vi "Ctrlr 2 Flag.vi"(8 "AutoArmIn":u8, 10 "Controller in":string, 11 "Enabled?":enum16{"Disabled", "Enabled"}(ring)) -> (0 "AutoArm Out":u8)   [LabVIEW 2012, in "BlockParty4150.lvrbt"]
uses:
  BlockParty4150.lvrbt
  <vilib>/NXT/Hardware/Plugins/Tetrix DC Motor/TetrixDCMotorAddress.ctl
  <vilib>/NXT/Hardware/Plugins/Tetrix 180 deg Servo/Tetrix180ServoAddress.ctl
  <vilib>/FTC/FTC Calculate Drive Power - Tank.vi
  <vilib>/NXT/NXTIO Xnodes/NXTIONodeSubVIs/TETRIX IO Move DC Motors.vi
  <vilib>/NXT/NXTIO Xnodes/NXTIONodeSubVIs/TETRIX IO Move Servos.vi
  <vilib>/NXT/NXTIO Xnodes/AddressXNode/NXTIOAddress.xnode
  <vilib>/NXT/Subs/LVHSConnector.ctl
  <vilib>/NXT/NXTIO Xnodes/NXTIOXNode/NXTIO.xnode
  <vilib>/NXT/LegoClasses/BrickReference/BrickReference.lvclass
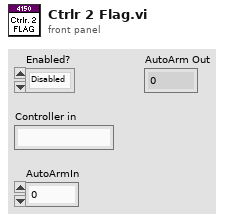
[diagram p1: front panel]
types:
  T1 = typedef "FTC ControllerState.ctl" = cluster{"Left X":i8, "Left Y":i8, "Right X":i8, "Right Y":i8, "Button Encoding 9-12":u8, "Button Encoding 1-8":u8, "POV":T2}
  T2 = typedef "FTC POVState.ctl" = i8
  T3 = typedef "FTC ButtonState.ctl" = cluster{"Button 1":bool, "Button 2":bool, "Button 3":bool, "Button 4":bool, "Button 5":bool, "Button 6":bool, "Button 7":bool, "Button 8":bool, "Button 9":bool, "Button 10":bool, "Button 11":bool, "Button 12":bool, "POV":T2}
  T4 = typedef "TetrixDCMotorAddress.ctl" = i32
  T5 = typedef "Tetrix180ServoAddress.ctl" = i32
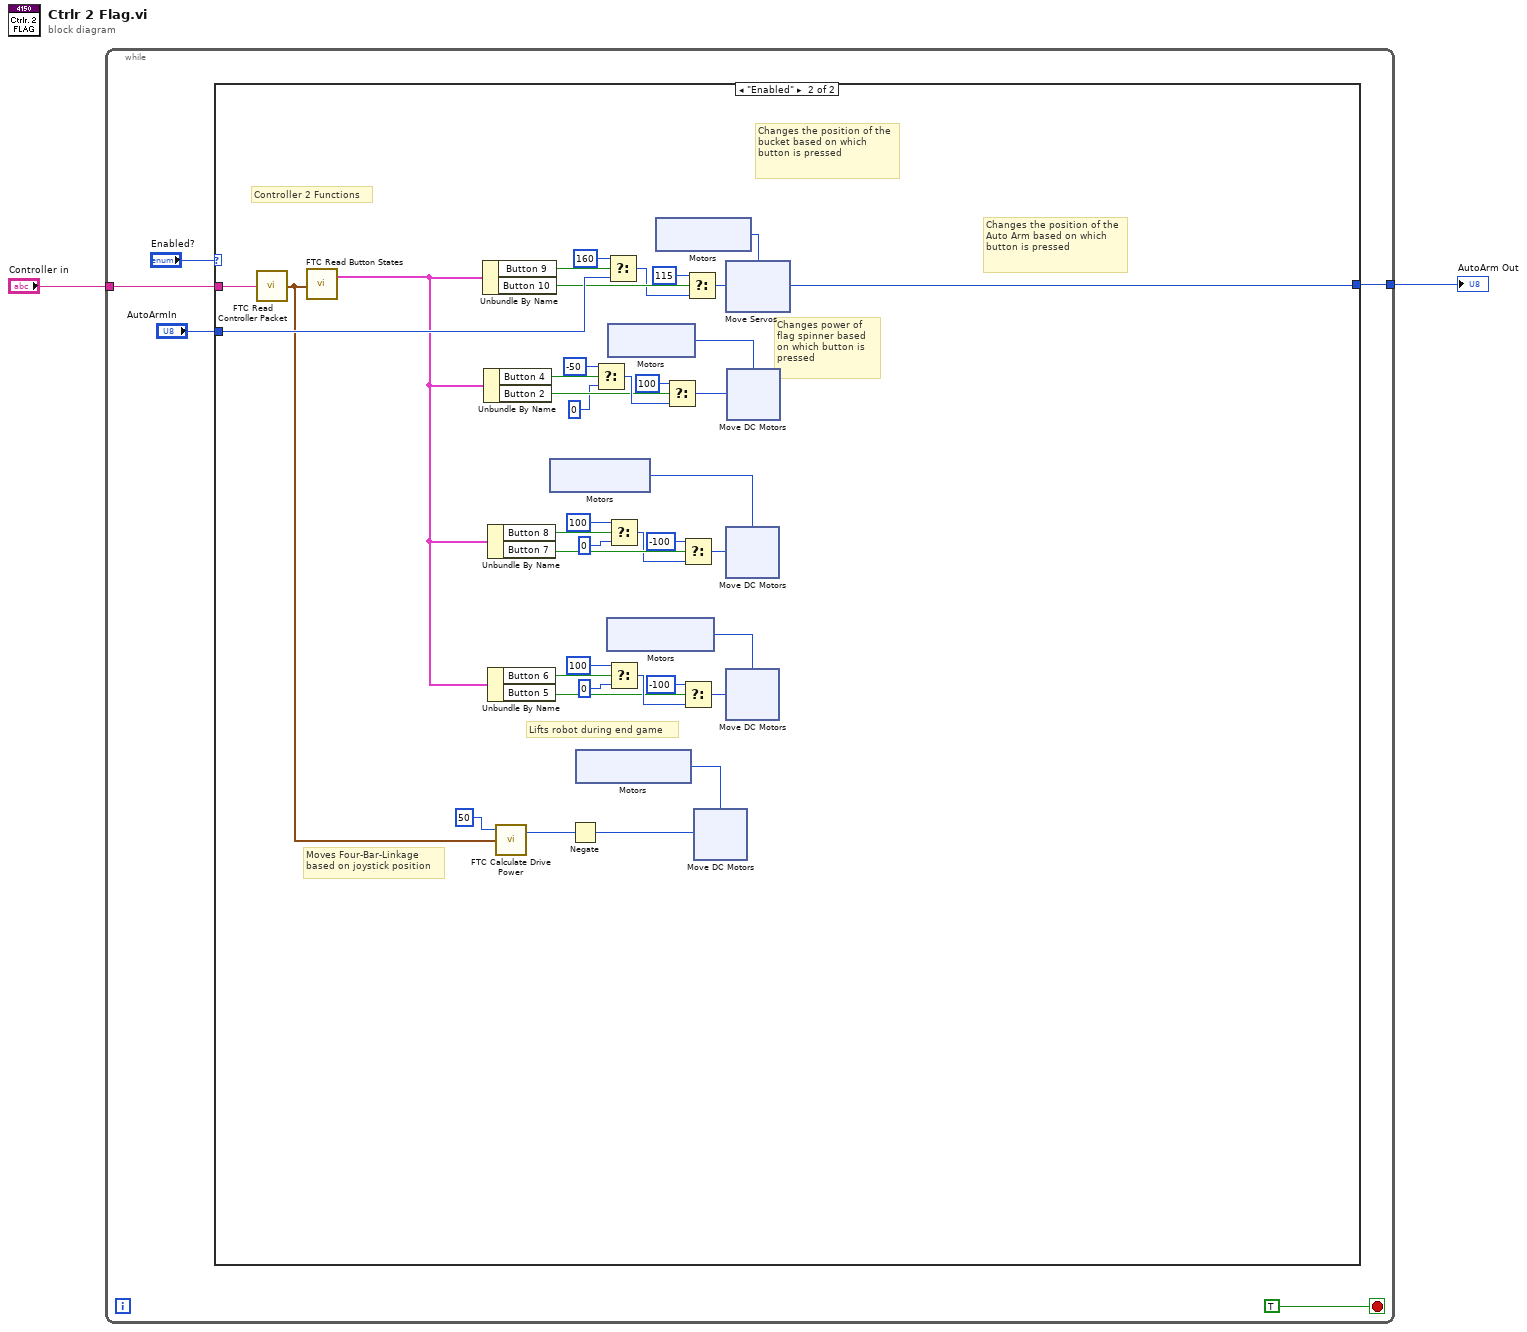
[diagram p0: block diagram]
diagram:
  n1 = while {
    tunnel: [w6] -> w2
    tunnel: "Controller in" -> [w4]
    stop <- TRUE stop-if-true
    n2 = case shown="\"Enabled\"" "Enabled?" {
      tunnel: w4 -> [_ w47]
      tunnel: "AutoArmIn" -> [w8 w46]
      tunnel: [w8 w45] -> w6
      frame "Disabled", Default {
      }
      frame "Enabled" {
        # "Changes the position of the bucket based on which button is pressed"
        # "Changes the position of the Auto Arm based on which button is pressed"
        # "Lifts robot during end game"
        # "Moves Four-Bar-Linkage\nbased on joystick position"
        # "Changes power of\nflag spinner based\non which button is \npressed"
        # "Controller 2 Functions"
        n3 = call <vilib>:"FTC Read Controller Packet.vi"("Packet"=w47) -> ("Controller State"=w21:T1)  [unwired: 4 in]
        n4 = call <vilib>:"FTC Read Button States.vi"("Controller State"=w21) -> ("Button States"=w11:T3)  [unwired: 2 in, 1 out]
        n5 = Unbundle By Name(w11) -> ("Button 9"=w41:bool, "Button 10"=w40:bool)
        n6 = Unbundle By Name(w11) -> ("Button 4"=w36:bool, "Button 2"=w35:bool)
        n7 = Unbundle By Name(w11) -> ("Button 8"=w30:bool, "Button 7"=w25:bool)
        n8 = Unbundle By Name(w11) -> ("Button 6"=w12:bool, "Button 5"=w16:bool)
        n9 = call-poly <vilib>:"FTC Calculate Drive Power.vi"("Controller State"=w21, "Power Level (50)"=i8 50) -> ("Left Motor Power"=w19:i8)  [unwired: 2 in, 1 out]
        n10 = xnode "Motors"() -> ("Motor"=w29:T4)
        n11 = Negate(x=w19) -> (-x=w18:i8)
        n12 = xnode "Motors"() -> ("Motor"=w44:T4)
        n13 = Select(t=i8 -50 ("Position 1"), s=w36, f=i8 0) -> (s? t:f=w37:i8)
        n14 = xnode "Motors"() -> ("Motor"=w9:T4)
        n15 = Select(t=u8 160 ("Position 1"), s=w41, f=w46) -> (s? t:f=w38:u8)
        n16 = xnode "Motors"() -> ("Motor"=w22:T4)
        n17 = Select(t=i8 100, s=w30, f=i8 0 ("Power/Speed 1")) -> (s? t:f=w24:i8)
        n18 = Select(t=i8 100, s=w12, f=i8 0 ("Power/Speed 1")) -> (s? t:f=w17:i8)
        n19 = xnode "Motors"() -> ("Motor"=w43:T5)
        n20 = Select(t=i8 100, s=w35, f=w37) -> (s? t:f=w31:i8)
        n21 = Select(t=i8 -100, s=w25, f=w24) -> (s? t:f=w23:i8)
        n22 = Select(t=i8 -100, s=w16, f=w17) -> (s? t:f=w10:i8)
        n23 = Select(t=u8 115 ("f"), s=w40, f=w38) -> (s? t:f=w45:u8)
        n24 = xnode "Move DC Motors"("Power/Speed 1"=w18, "Motors"=w44) -> ()  [unwired: 1 in, 1 out]
        n25 = xnode "Move Servos"("Position 1"=w45, "Motors"=w43) -> ()  [unwired: 1 in, 1 out]
        n26 = xnode "Move DC Motors"("Power/Speed 1"=w23, "Motors"=w29) -> ()  [unwired: 1 in, 1 out]
        n27 = xnode "Move DC Motors"("Power/Speed 1"=w10, "Motors"=w9) -> ()  [unwired: 1 in, 1 out]
        n28 = xnode "Move DC Motors"("Power/Speed 1"=w31, "Motors"=w22) -> ()  [unwired: 1 in, 1 out]
      }
    }
  }
  "AutoArm Out" <- w2
